vi "Handle Exit.vi"(8 "error in (no error)":errorcluster, 9 "Stop Argument":T1, 10 "Admin in":refnum<class "Delacor_lib_QMH_Module Admin.lvclass">, 11 "VI reference":refnum<vi>) -> (0 "error out":errorcluster, 3 "Wait for Module to stop?":bool)   [LabVIEW 2015, in "TestStand Manager_DQMH.lvlib"]
doc: "This VI handles the Exit Message for a DQMH Singleton module. \n\nThis VI determines if the message was received via the Stop Request or not. If the Exit message was received via the Request Event to Stop the module then there is no need to send the Stop Request again. If it was not, then the Stop Request needs to be fired so the Event Handling Loop can stop.\n\nThis VI also hides the Main.vi Front Panel, this is to ensure that the module stays in memory until the very last step in the Main.vi which is to close the front panel.\n_____\nBased on Delacor QMH Project Template 2.0.0.62.\n\n<b>Note:</b> This VI was modified by the <b>Validate DQMH Module</b> tool to upgrade it to use an improved error handling scheme, where the FP.Open method will not manipulate the error stream through this VI.\n____\nDelacor QMH Thermal Chamber Examples 4.0.0.21\nCopyright (c) 2018, Delacor"
uses:
  TestStand Manager_DQMH.lvlib
  <vilib>/Delacor/Delacor QMH/Libraries/Module Admin_class/Delacor_lib_QMH_Module Admin.lvclass
  Stop Argument--cluster.ctl
  <vilib>/Delacor/Delacor QMH/Libraries/Module Admin_class/Delacor_lib_QMH_Module Admin.lvclass/Delacor_lib_QMH_Module Admin.ctl
  <vilib>/Delacor/Delacor QMH/Libraries/Module Admin_class/Delacor_lib_QMH_Get External Launch.vi
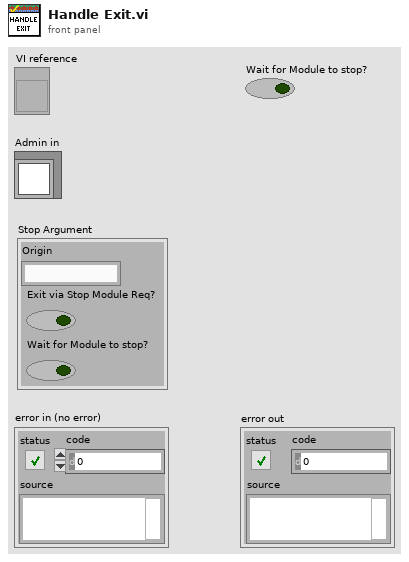
[diagram p1: front panel]
types:
  T1 = typedef "TestStand Manager_DQMH.lvlib/Stop Argument--cluster.ctl" = cluster{"Origin":string, "Exit via Stop Module Req?":bool, "Wait for Module to stop?":bool}
  T2 = enum32{"Invalid", "Standard", "Closed", "Hidden", "Minimized", "Maximized"}
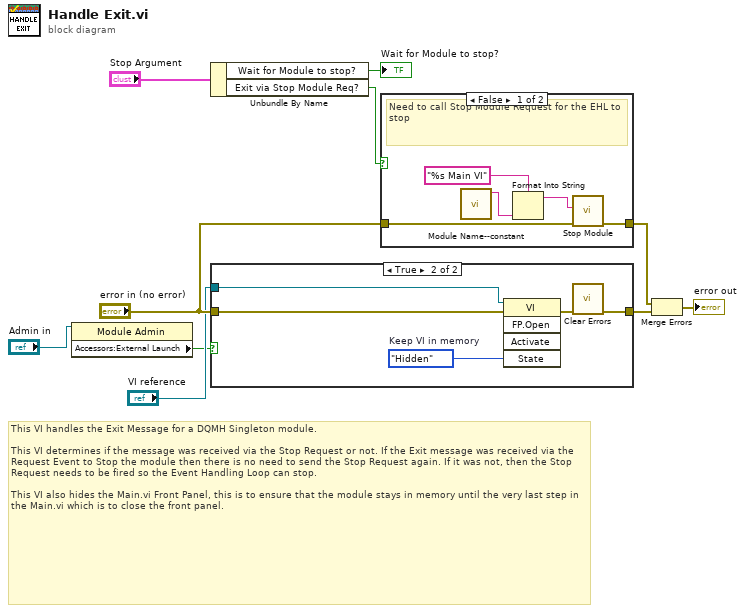
[diagram p0: block diagram]
diagram:
  # "This VI handles the Exit Message for a DQMH Singleton module. \n\nThis VI determines if the message was received via the Stop Request or not. If the Exit message was received via the Request Event to Stop the module then there is no need to send the Stop Request again. If it was not, then the Stop Request needs to be fired so the Event Handling Loop can stop.\n\nThis VI also hides the Main.vi Front Panel, this is to ensure that the module stays in memory until the very last step in the Main.vi which is to close the front panel."
  n1 = property class="Module Admin"(reference="Admin in") -> ("Accessors:External Launch"=w3:bool)  [unwired: 1 in, 2 out]
  n2 = Unbundle By Name("Stop Argument") -> ("Wait for Module to stop?"=→"Wait for Module to stop?":bool, "Exit via Stop Module Req?"=w5:bool)
  n3 = case shown="True" w3 {
    tunnel: "VI reference" -> [_ w16]
    tunnel: [w11 w12] -> w1
    tunnel: "error in (no error)" -> [w11 w14]
    frame False {
    }
    frame True {
      w13 = T2."Hidden"  # Keep VI in memory
      n4 = invoke class="VI" method="FP.Open"(reference=w16, error in=w14, "State"=w13) -> (error out=w15:errorcluster)  [unwired: 2 in, 4 out]
      n5 = call <vilib>:"Clear Errors.vi"("error in (no error)"=w15) -> ("error out"=w12:errorcluster)  [unwired: 5 in, 1 out]
    }
  }
  n6 = case "Exit came from Stop Module Request?" shown="False" w5 {
    tunnel: [w19 w22] -> w7
    tunnel: "error in (no error)" -> [w17 w22]
    frame False {
      # "Need to call Stop Module Request for the EHL to stop"
      n7 = call "Module Name--constant.vi"() -> ("Module Name"=w18:string)  [unwired: 11 in]
      n8 = Format Into String(format string="%s Main VI", w18) -> (resulting string=w20:string)  [unwired: 2 in, 1 out]
      n9 = call "Stop Module.vi"("error in (no error)"=w17, "Origin"=w20) -> ("error out"=w19:errorcluster)  [unwired: 9 in]
    }
    frame True {
      # "no need to call Stop Module Request again."
    }
  }
  n10 = Merge Errors(w7, w1) -> (→"error out":errorcluster)
